vi "get_number_of_channels.vi"(8 "error in (no error)":errorcluster, 11 "GenericImageProcessor.lvclass in":refnum<class "GenericImageProcessor.lvclass">) -> (0 "error out":errorcluster, 2 "number of channels":i32, 3 "GenericImageProcessor.lvclass out":refnum<class "GenericImageProcessor.lvclass">)   [LabVIEW 2010, in "GenericImageProcessor.lvclass"]
uses:
  GenericImageProcessor.lvclass
  GenericImageProcessor.lvclass/GenericImageProcessor.ctl
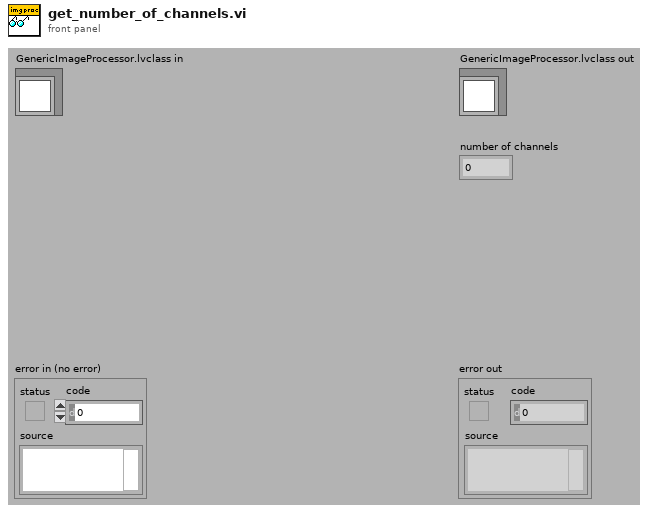
[diagram p1: front panel]
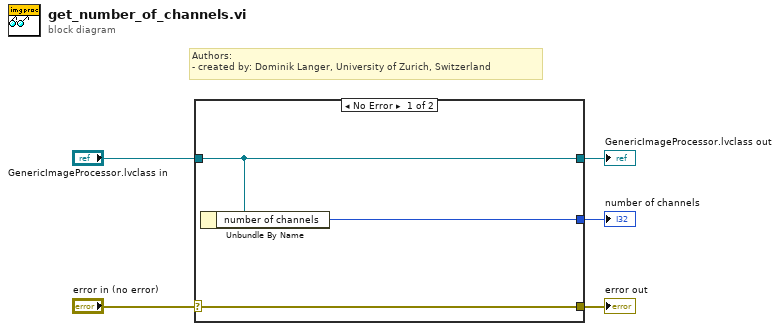
[diagram p0: block diagram]
diagram:
  # "Authors: \n- created by: Dominik Langer, University of Zurich, Switzerland"
  n1 = case shown="No Error" "error in (no error)" {
    selector: "error in (no error)" -> [w8 w9]
    tunnel: [w8 w9] -> w4
    tunnel: [w7 w10] -> w2
    tunnel: "GenericImageProcessor.lvclass in" -> [w7 w10]
    tunnel: [w6 _] -> w1
    frame No Error {
      n2 = Unbundle By Name(w7) -> ("number of channels"=w6:i32)
    }
    frame Error {
    }
  }
  "error out" <- w4
  "GenericImageProcessor.lvclass out" <- w2
  "number of channels" <- w1
